vi "create Freeform Scan Pattern.vi"(2 "Apodization?":bool, 3 "positions":sgl[](array[numeric]), 4 "error in (no error)":errorcluster, 5 "Probe":refnum<class "Probe.lvclass">, 6 "SizeY":u32, 7 "SizeX":u32) -> (0 "error out":errorcluster, 1 "Scan Pattern":refnum<class "Scan Pattern.lvclass">)   [LabVIEW 2018]
uses:
  SpectralRadar/LabVIEW/2012/user.lib/SpectralRadar.llb/Scan Pattern.lvclass
  SpectralRadar/LabVIEW/2012/user.lib/SpectralRadar.llb/Probe.lvclass
  <vilib>/Utility/error.llb/Error Cluster From Error Code.vi
  <vilib>/ErrorRing/Error Ring.xnode
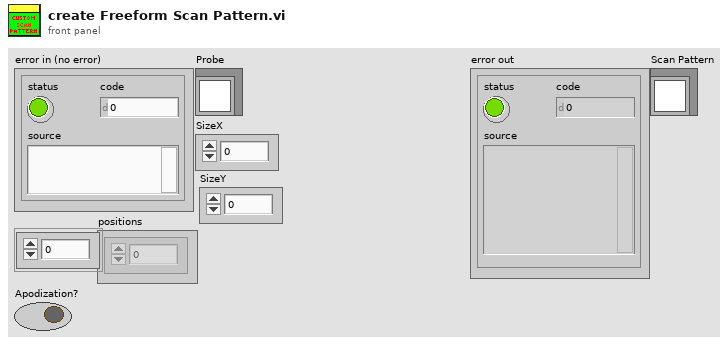
[diagram p1: front panel]
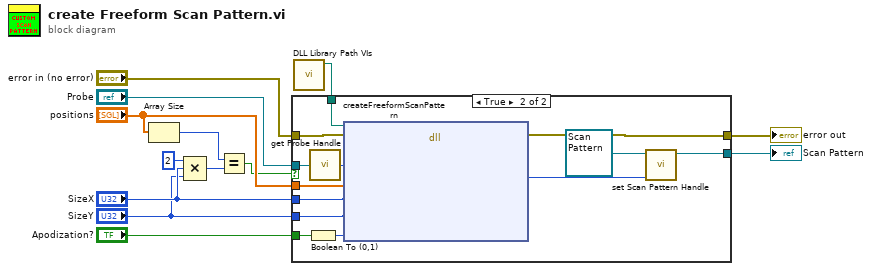
[diagram p0: block diagram]
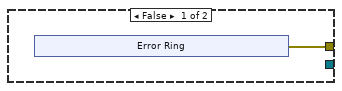
[diagram p2: hidden frame]
diagram:
  n1 = Array Size(array="positions") -> (size(s)=w3:i32)
  n2 = Compound Arithmetic op=MULTIPLY(u32 2 ("value"), "SizeX", "SizeY") -> (w4:u32)
  n3 = Equal?(x=w3, y=w4) -> (x = y?=w2:bool)
  n4 = call "DLL Library Path VIs.vi"() -> ("SpectralRadarDLL"=w1:path)  [unwired: 8 in, 3 out]
  n5 = case shown="True" w2 {
    tunnel: "error in (no error)" -> [_ w32]
    tunnel: [w14 w31] -> w12
    tunnel: [_ w29] -> w11
    tunnel: "Probe" -> [_ w27]
    tunnel: "positions" -> [_ w25]
    tunnel: "SizeX" -> [_ w24]
    tunnel: "SizeY" -> [_ w23]
    tunnel: "Apodization?" -> [_ w21]
    tunnel: w1 -> [_ w20]
    frame False {
      n6 = xnode "Error Ring"() -> ("error out"=w14:errorcluster)
    }
    frame True {
      n7 = Boolean To (0,1)(Boolean=w21) -> (0, 1=w22:i16)
      n8 = call "get Probe Handle.vi"("GalvoControl"=w27) -> ("Galvo Control Handle"=w26:u64)
      n9 = dll-call lib="C:/Project/SerialSectOCT - FFT GPU/SerialSectOCT/Labview Software/DLL/SpectralRadar.dll" fn="createFreeformScanPattern"(path in=w20, error in=w32, "ProbeHandle"=w26, "positions"=w25, "SizeX"=w24, "SizeY"=w23, "Apodization"=w22) -> (error out=w31:errorcluster, "ScanPatternHandle"=w30:u64)  [unwired: 6 in, 1 out]
      n10 = call "set Scan Pattern Handle.vi"("Handle"=w30, "Scan Pattern"=refnum<class "Scan Pattern.lvclass"> refnum) -> ("Scan Pattern"=w29:refnum<class "Scan Pattern.lvclass">)  [unwired: 5 in]
    }
  }
  "error out" <- w12
  "Scan Pattern" <- w11
